vi "TurnToAngle.vi"() -> ()   [LabVIEW 2017]
uses:
  Framework/Robot Global Data.vi
panel:
  in  "Angle":dbl
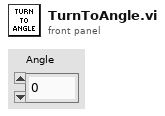
[diagram p1: front panel]
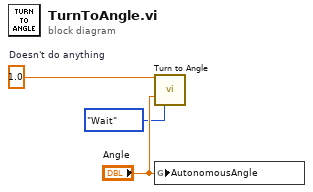
[diagram p0: block diagram]
diagram:
  w1 = 1.0  # Doesn't do anything
  n1 = call "Turn to Angle.vi"("Speed"=w1, "Target Angle"="Angle", "Synchronication"=enum16{"Start", "Wait"}."Wait") -> ()  [unwired: 12 in, 1 out]
  n2 = global write "Robot Global Data.vi" "AutonomousAngle"("Angle") -> ()
